vi "Simulate CE14 data (SubVI).vi"(8 "freq":dbl=50.06 format="%#_13g", 9 "pf":dbl=0.997 format="%#_13g", 10 "ACI":dbl=180.0 format="%#_13g", 11 "ACV":dbl=220.08 format="%#_13g") -> (3 "Array":T1[](array[typedef]))   [LabVIEW 2018, in "CE14_v2.lvlib"]
uses:
  Instrument Drivers/LVdriver_CE14(eMIC)/type defs/CE14.data.ctl
  CE14_v2.lvlib
  Instrument Drivers/LVdriver_CE14(eMIC)/CE14_eMIC.lvlib
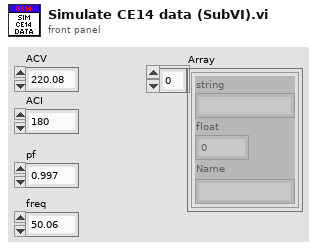
[diagram p1: front panel]
types:
  T1 = typedef "CE14_eMIC.lvlib/CE14.data.ctl" = cluster{"string":string, "float":dbl, "Name":string}
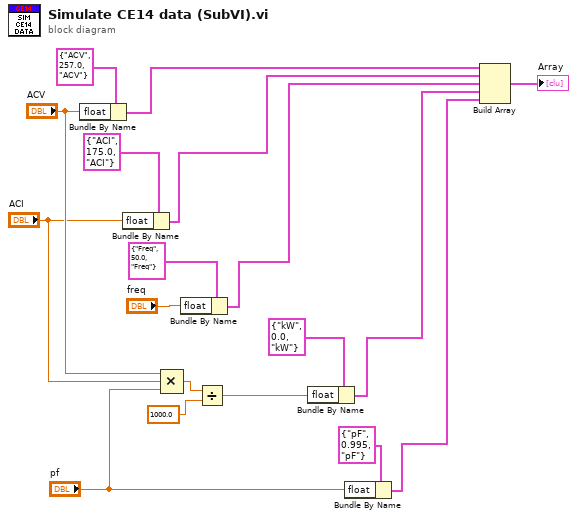
[diagram p0: block diagram]
diagram:
  n1 = Bundle By Name(cluster=T1 {"string"="ACV", "float"=257.0, "Name"="ACV"} ("data out"), "float"="ACV") -> (w16:T1)
  n2 = Bundle By Name(cluster=T1 {"string"="ACI", "float"=175.0, "Name"="ACI"} ("data out"), "float"="ACI") -> (w14:T1)
  n3 = Compound Arithmetic op=MULTIPLY("ACV", "ACI", "pf") -> (w3:dbl)
  n4 = Bundle By Name(cluster=T1 {"string"="Freq", "float"=50.0, "Name"="Freq"} ("data out"), "float"="freq") -> (w11:T1)
  n5 = Divide(x=w3, y=1000.0) -> (x/y=w1:dbl)
  n6 = Bundle By Name(cluster=T1 {"string"="kW", "float"=0.0, "Name"="kW"} ("data out"), "float"=w1) -> (w9:T1)
  n7 = Bundle By Name(cluster=T1 {"string"="pF", "float"=0.995, "Name"="pF"} ("data out"), "float"="pf") -> (w7:T1)
  n8 = Build Array(w16, w14, w11, w9, w7) -> (→"Array":T1[])
